vi "API - Update Rx Channel Order.vi"(6 "Channel Names":string[](array[string]), 8 "error in (no error)":errorcluster, 11 "Node Ptr":T1 format="%.0x") -> (0 "error out":errorcluster, 3 "Node Ptr out":T1 format="%.0x")   [LabVIEW 2016, in "UDP-Custom-Device System Explorer.lvlib"]
uses:
  UDP-Custom-Device System Explorer.lvlib
  <vilib>/NI Veristand/Custom Device API/Custom Device Item Ref.ctl
  Shared/Constants.vi
  <vilib>/NI VeriStand/Custom Device API/Custom Device API.lvlib
  Shared/UDP-Custom-Device Shared.lvlib
  <vilib>/NI VeriStand/Custom Device Tools/Custom Device Utility Library/Custom Device Utility Library.lvlib
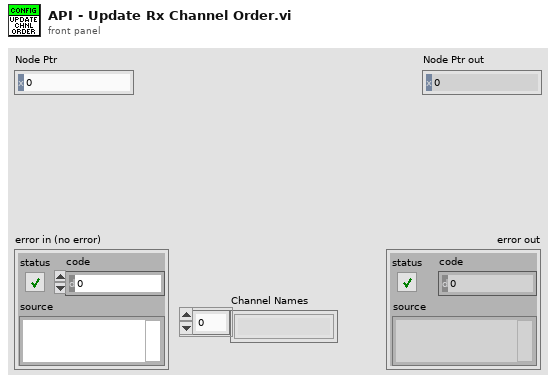
[diagram p1: front panel]
types:
  T1 = typedef "Custom Device API.lvlib/Custom Device Item Ref.ctl" = u64
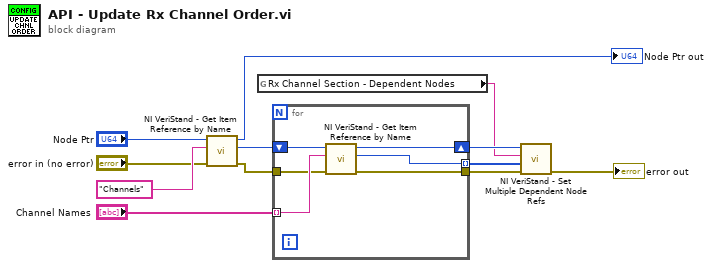
[diagram p0: block diagram]
diagram:
  n1 = call <vilib>:"NI VeriStand - Get Item Reference by Name.vi"("error in (no error)"="error in (no error)", "Item Name"="Channels" ("Section Name"), "Parent Ref in"="Node Ptr") -> ("error out"=w4:errorcluster, "Item Ref"=w9:T1, "Parent Ref out"=→"Node Ptr out":T1)  [unwired: 5 in, 1 out]
  n2 = global read "Constants.vi" "Rx Channel Section - Dependent Nodes"() -> (w5:string)
  n3 = for {
    tunnel: "Channel Names" -> [w17] mode=indexing
    tunnel: [w16] -> w6 mode=indexing
    tunnel: w4 -> [w14]
    shift-right: [w15] -> w7
    shift-left: w9 -> [w18]
    tunnel: [w13] -> w3
    n4 = call <vilib>:"NI VeriStand - Get Item Reference by Name.vi"("error in (no error)"=w14, "Item Name"=w17, "Parent Ref in"=w18) -> ("error out"=w13:errorcluster, "Item Ref"=w16:T1, "Parent Ref out"=w15:T1)  [unwired: 5 in, 1 out]
  }
  n5 = call <vilib>:"NI VeriStand - Set Multiple Dependent Node Refs.vi"("error in (no error)"=w3, "Dependent Node Refs"=w6, "Base Property Name"=w5, "Item Ref in"=w7) -> ("error out"=→"error out":errorcluster)  [unwired: 6 in, 1 out]
